vi "mutiple dry pump control(1).vi"() -> ()   [LabVIEW 2020]
uses:
  <vilib>/Instr/_visa.llb/VISA Configure Serial Port (Instr).vi
panel:
  out "overheat 2":bool
  out "overheat":bool
  out "T2":dbl(graph)
  out "T1":dbl(graph)
  in  "VISA resource name":refnum<visa-resource-name>
  in  "stop":bool
  in  "Auto":bool
  out "T2":dbl(knob) scale=0.0..150.0
  out "Temperature of Pump 2":dbl
  out "T1":dbl(knob) scale=0.0..150.0
  out "Temperature of Pump 1":dbl
  in  "Set the address":bool
  in  "Set the address(0 to stop mutiple control)":dbl
  in  "Turn off the pump":bool
  in  "pump number":dbl
  in  "Turn on the pump":bool
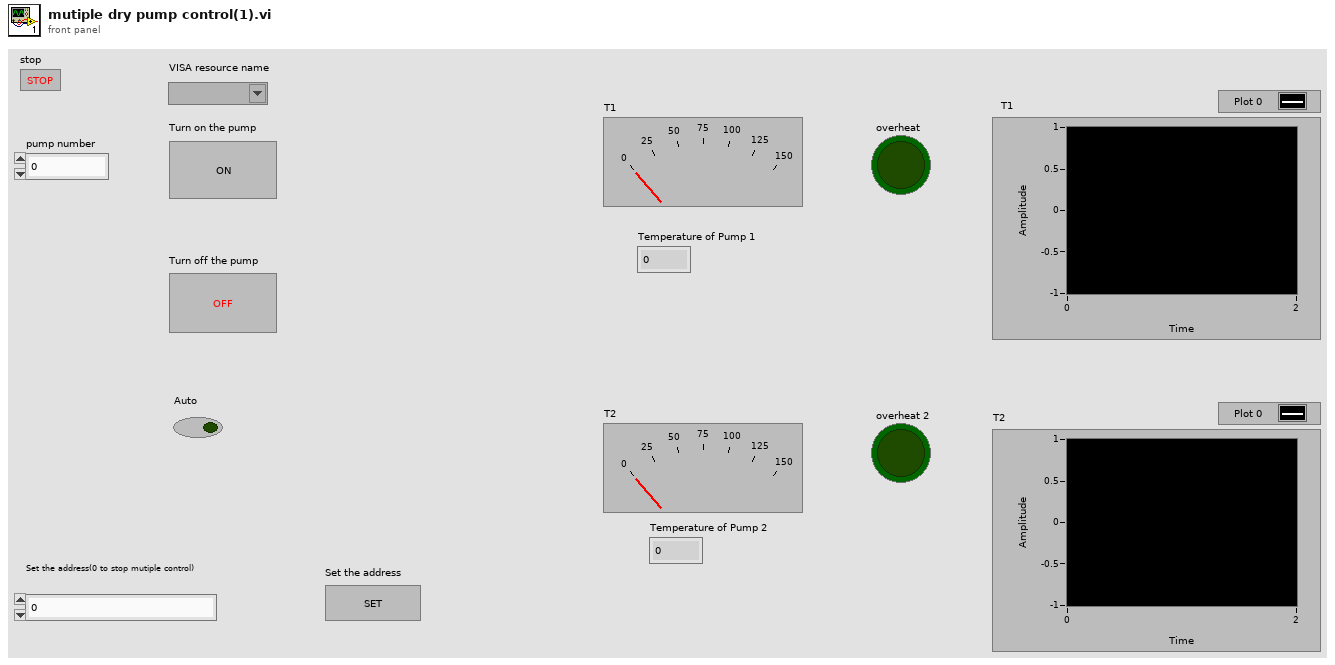
[diagram p1: front panel]
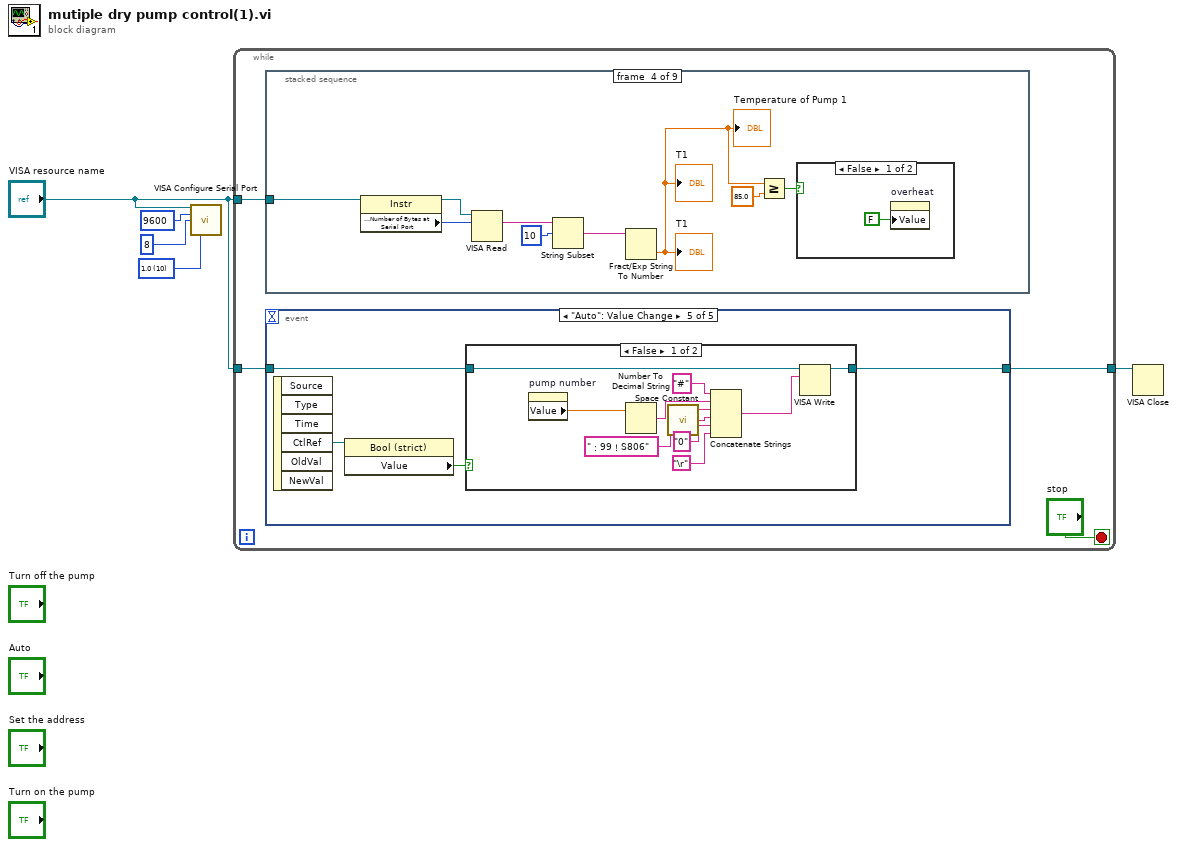
[diagram p0: block diagram]
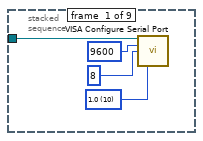
[diagram p2: hidden frame]
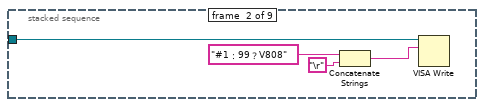
[diagram p3: hidden frame]
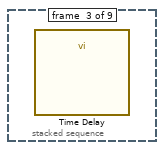
[diagram p4: hidden frame]
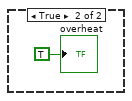
[diagram p5: hidden frame]
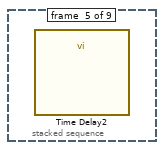
[diagram p6: hidden frame]
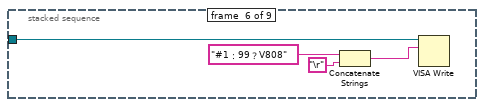
[diagram p7: hidden frame]
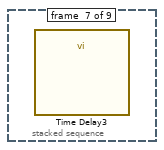
[diagram p8: hidden frame]
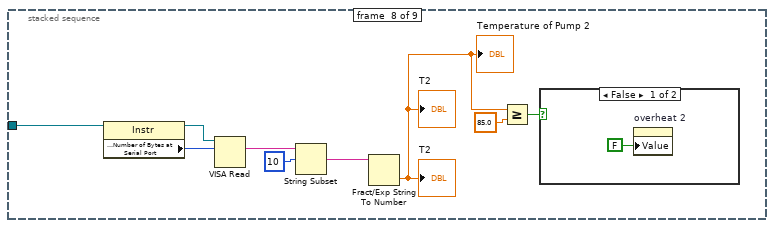
[diagram p9: hidden frame]
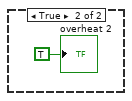
[diagram p10: hidden frame]
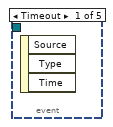
[diagram p12: hidden frame]
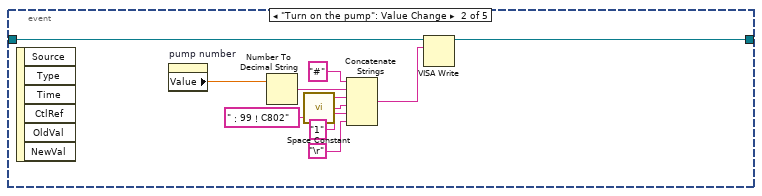
[diagram p13: hidden frame]
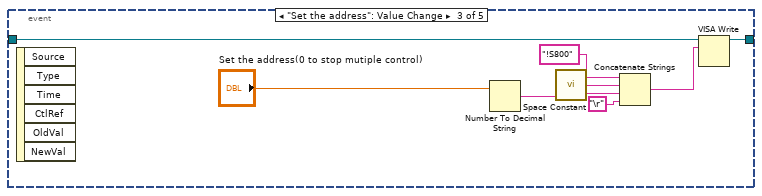
[diagram p14: hidden frame]
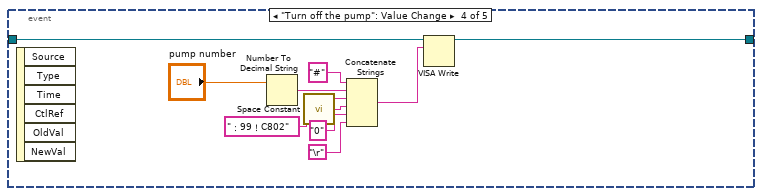
[diagram p15: hidden frame]
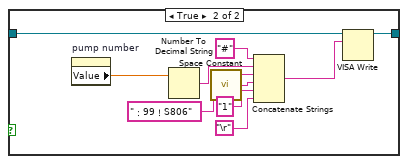
[diagram p16: hidden frame]
diagram:
  w3 = u16 10 items=["1.0"=10, "1.5"=15, "2.0"=20] ("stop bits (10: 1 bit)")
  n1 = call-poly "VISA Configure Serial Port"("VISA resource name"="VISA resource name", "baud rate (9600)"=u32 9600, "data bits (8)"=u16 8, "stop bits (10: 1 bit)"=w3) -> ()  [unwired: 10 in, 2 out]
  n2 = while {
    tunnel: "VISA resource name" -> [w8]
    tunnel: [w7] -> w2
    tunnel: "VISA resource name" -> [w6]
    stop <- "stop" stop-if-true
    n3 = stacked-sequence {
      tunnel: w6 -> [w10 w14 _ w25 _ w29 _ w37 _]
      frame #0 {
        w11 = u16 10 items=["1.0"=10, "1.5"=15, "2.0"=20] ("stop bits (10: 1 bit)")
        n4 = call-poly "VISA Configure Serial Port"("VISA resource name"=w10, "baud rate (9600)"=u32 9600, "data bits (8)"=u16 8, "stop bits (10: 1 bit)"=w11) -> ()  [unwired: 10 in, 2 out]
      }
      frame #1 {
        n5 = Concatenate Strings("#1：99？V808", "\r") -> (w15:string)
        n6 = VISA Write(VISA resource name=w14, write buffer=w15) -> ()  [unwired: 1 in, 3 out]
      }
      frame #2 {
        n7 = call "Time Delay"() -> ()  [unwired: 11 in, 1 out]
      }
      frame #3 {
        n8 = property class="Instr"(reference=w25) -> (reference out=w26:refnum<visa-resource-name>, "Serial Settings:Number of Bytes at Serial Port"=w18:u32)  [unwired: 1 in, 1 out]
        n9 = VISA Read(VISA resource name=w26, byte count=w18) -> (read buffer=w24:string)  [unwired: 1 in, 3 out]
        n10 = String Subset(string=w24, offset (0)=10) -> (substring=w22:string)  [unwired: 1 in]
        n11 = Fract/Exp String To Number(string=w22) -> (number=w21:dbl)  [unwired: 3 in, 1 out]
        "T1" <- w21
        "T1" <- w21
        "Temperature of Pump 1" <- w21
        n12 = Greater Or Equal?(x=w21, y=85.0) -> (x >= y?=w19:bool)
        n13 = case shown="False" w19 {
          frame False {
            n14 = property on="overheat" class="Bool (strict)"("Value"=FALSE ("overheat")) -> ()  [unwired: 2 in, 2 out]
          }
          frame True {
            "overheat" <- TRUE ("overheat")
          }
        }
      }
      frame #4 {
        n15 = call "Time Delay2"() -> ()  [unwired: 11 in, 1 out]
      }
      frame #5 {
        n16 = Concatenate Strings("#1：99？V808", "\r") -> (w30:string)
        n17 = VISA Write(VISA resource name=w29, write buffer=w30) -> ()  [unwired: 1 in, 3 out]
      }
      frame #6 {
        n18 = call "Time Delay3"() -> ()  [unwired: 11 in, 1 out]
      }
      frame #7 {
        n19 = property class="Instr"(reference=w37) -> (reference out=w41:refnum<visa-resource-name>, "Serial Settings:Number of Bytes at Serial Port"=w33:u32)  [unwired: 1 in, 1 out]
        n20 = VISA Read(VISA resource name=w41, byte count=w33) -> (read buffer=w40:string)  [unwired: 1 in, 3 out]
        n21 = String Subset(string=w40, offset (0)=10) -> (substring=w38:string)  [unwired: 1 in]
        n22 = Fract/Exp String To Number(string=w38) -> (number=w34:dbl)  [unwired: 3 in, 1 out]
        "T2" <- w34
        "T2" <- w34
        "Temperature of Pump 2" <- w34
        n23 = Greater Or Equal?(x=w34, y=85.0) -> (x >= y?=w35:bool)
        n24 = case shown="False" w35 {
          frame False {
            n25 = property on="overheat 2" class="Bool (strict)"("Value"=FALSE ("overheat 2")) -> ()  [unwired: 2 in, 2 out]
          }
          frame True {
            "overheat 2" <- TRUE ("overheat 2")
          }
        }
      }
      frame #8 {
      }
    }
    n26 = event shown="[4] \"Auto\": Value Change" {
      selector: _ -> [_ _ _ _ _]
      dyn-events: _ -> [_ _ _ _ _]
      timeout: _ -> [_ _ _ _ _]
      tunnel: w8 -> [_ w45 w56 w63 w73]
      tunnel: [_ w44 w55 w62 w72] -> w7
      event Timeout {
        n27 = event-data() -> ()  [unwired: 1 in, 3 out]
      }
      event "Turn on the pump": Value Change {
        n28 = event-data() -> ()  [unwired: 1 in, 6 out]
        n29 = property on="pump number" class="DigNum (strict)"() -> ("Value"=w53:dbl)  [unwired: 2 in, 2 out]
        n30 = Number To Decimal String(number=w53) -> (decimal integer string=w52:string)  [unwired: 1 in]
        n31 = call <vilib>:"Space Constant.vi"() -> ("String"=w49:string)
        n32 = Concatenate Strings("#", w52, "：99！C802", w49, "1", "\r") -> (w46:string)
        n33 = VISA Write(VISA resource name=w45, write buffer=w46) -> (VISA resource name out=w44:refnum<visa-resource-name>)  [unwired: 1 in, 2 out]
      }
      event "Set the address": Value Change {
        n34 = event-data() -> ()  [unwired: 1 in, 6 out]
        n35 = Number To Decimal String(number="Set the address(0 to stop mutiple control)") -> (decimal integer string=w58:string)  [unwired: 1 in]
        n36 = call <vilib>:"Space Constant.vi"() -> ("String"=w59:string)
        n37 = Concatenate Strings("!S800", w59, w58, "\r") -> (w57:string)
        n38 = VISA Write(VISA resource name=w56, write buffer=w57) -> (VISA resource name out=w55:refnum<visa-resource-name>)  [unwired: 1 in, 2 out]
      }
      event "Turn off the pump": Value Change {
        n39 = event-data() -> ()  [unwired: 1 in, 6 out]
        n40 = Number To Decimal String(number="pump number") -> (decimal integer string=w71:string)  [unwired: 1 in]
        n41 = call <vilib>:"Space Constant.vi"() -> ("String"=w68:string)
        n42 = Concatenate Strings("#", w71, "：99！C802", w68, "0", "\r") -> (w65:string)
        n43 = VISA Write(VISA resource name=w63, write buffer=w65) -> (VISA resource name out=w62:refnum<visa-resource-name>)  [unwired: 1 in, 2 out]
      }
      event "Auto": Value Change {
        n44 = event-data() -> ("CtlRef"=w75:refnum<vi>)  [unwired: 1 in, 5 out]
        n45 = property class="Bool (strict)"(reference=w75) -> ("Value"=w74:bool)  [unwired: 1 in, 2 out]
        n46 = case shown="False" w74 {
          tunnel: w73 -> [w77 w87]
          tunnel: [w76 w86] -> w72
          frame False {
            n47 = property on="pump number" class="DigNum (strict)"() -> ("Value"=w78:dbl)  [unwired: 2 in, 2 out]
            n48 = Number To Decimal String(number=w78) -> (decimal integer string=w85:string)  [unwired: 1 in]
            n49 = call <vilib>:"Space Constant.vi"() -> ("String"=w82:string)
            n50 = Concatenate Strings("#", w85, "：99！S806", w82, "0", "\r") -> (w79:string)
            n51 = VISA Write(VISA resource name=w77, write buffer=w79) -> (VISA resource name out=w76:refnum<visa-resource-name>)  [unwired: 1 in, 2 out]
          }
          frame True {
            n52 = property on="pump number" class="DigNum (strict)"() -> ("Value"=w88:dbl)  [unwired: 2 in, 2 out]
            n53 = Number To Decimal String(number=w88) -> (decimal integer string=w95:string)  [unwired: 1 in]
            n54 = call <vilib>:"Space Constant.vi"() -> ("String"=w92:string)
            n55 = Concatenate Strings("#", w95, "：99！S806", w92, "1", "\r") -> (w89:string)
            n56 = VISA Write(VISA resource name=w87, write buffer=w89) -> (VISA resource name out=w86:refnum<visa-resource-name>)  [unwired: 1 in, 2 out]
          }
        }
      }
    }
  }
  n57 = VISA Close(VISA resource name=w2) -> ()  [unwired: 1 in, 1 out]
